vi "CallByRefParallel.vi"(6 "Auto Dispose Ref":bool=TRUE, 8 "error in (no error)":errorcluster, 9 "Control values":variant[](array[variant]), 10 "Control names":string[](array[string]), 11 "VI Refnum":refnum<vi>) -> (0 "error out":errorcluster, 3 "VI Refnum dup":refnum<vi>)   [LabVIEW 2011, in "COSYLib.lvlib"]
doc: "Utility VI for calling a VI by reference *in parallel*. It is a simple wrapper around a series of \"Set Control Value\" (Ctrl Val.Set) and \"Run\" calls, mainly intended to save space on a BD.\n\nSet <B>Auto Dispose Ref</B> to FALSE if you want to manage the reference to the VI yourself. If TRUE (default), the ownership of reference is passed on the target VI (see the LabVIEW help).\n\nIf the target VI is already running, nothing is done (no FP controls are set) and an error is returned."
uses:
  COSYLib.lvlib
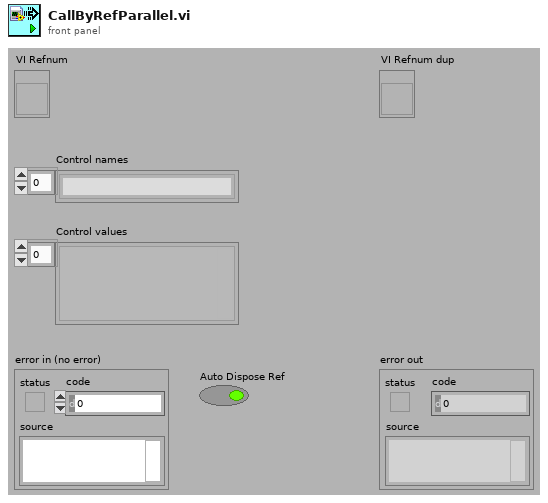
[diagram p1: front panel]
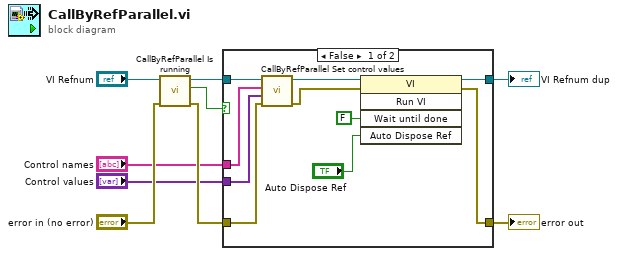
[diagram p0: block diagram]
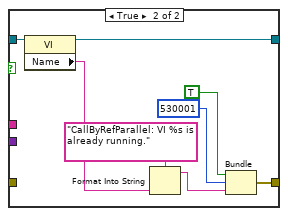
[diagram p2: hidden frame]
diagram:
  n1 = call "CallByRefParallel Is running.vi"("error in (no error)"="error in (no error)", "VI Refnum"="VI Refnum") -> ("error out"=w8:errorcluster, "Is running?"=w1:bool, "VI Refnum dup"=w2:refnum<vi>)  [unwired: 7 in]
  n2 = case shown="False" w1 {
    tunnel: [w18 w22] -> w7
    tunnel: [w17 w27] -> w6
    tunnel: w2 -> [w15 w23]
    tunnel: "Control names" -> [w14 _]
    tunnel: "Control values" -> [w13 _]
    tunnel: w8 -> [w12 _]
    frame False {
      n3 = call "CallByRefParallel Set control values.vi"("error in (no error)"=w12, "Control values"=w13, "Control names"=w14, "VI Refnum"=w15) -> ("error out"=w10:errorcluster, "VI Refnum dup"=w11:refnum<vi>)  [unwired: 6 in]
      n4 = invoke class="VI" method="Run VI"(reference=w11, error in=w10, "Wait until done"=FALSE ("Wait Until Done"), "Auto Dispose Ref"="Auto Dispose Ref") -> (reference out=w18:refnum<vi>, error out=w17:errorcluster)  [unwired: 1 in, 3 out]
    }
    frame True {
      n5 = property class="VI"(reference=w23) -> (reference out=w22:refnum<vi>, "Name"=w21:string)  [unwired: 1 in, 1 out]
      n6 = Format Into String(format string="CallByRefParallel: VI %s is already running." ("source"), w21) -> (resulting string=w24:string)  [unwired: 2 in, 1 out]
      n7 = Bundle("status"=TRUE, "code"=530001, w24) -> (w27:cluster{"status":bool, "code":i32, string})  [unwired: 1 in]
    }
  }
  "error out" <- w6
  "VI Refnum dup" <- w7
